vi "Read Data.vi"(3 "Error In":errorcluster) -> (0 "error out":errorcluster, 1 "text":string, 2 "appended path":path)   [LabVIEW 2017]
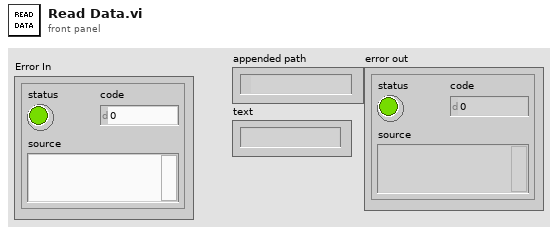
[diagram p1: front panel]
types:
  T1 = enum16{"open", "replace", "create", "open or create", "replace or create", "replace or create with confirmation"}
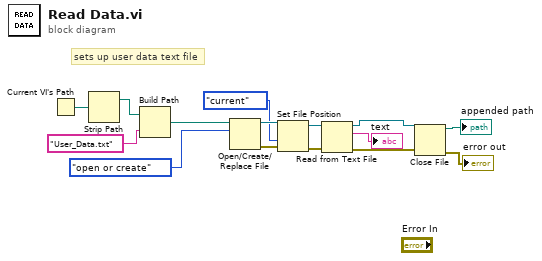
[diagram p0: block diagram]
diagram:
  # "sets up user data text file"
  n1 = Current VI's Path() -> (path=w8:path)
  n2 = Strip Path(path=w8) -> (stripped path=w14:path)  [unwired: 1 out]
  n3 = Build Path(base path=w14, name or relative path="User_Data.txt") -> (appended path=w12:path)
  n4 = Open/Create/Replace File(file path (use dialog)=w12, operation (0:open)=T1."open or create") -> (refnum out=w10:refnum<file>, error out=w11:errorcluster)  [unwired: 4 in, 1 out]
  n5 = Set File Position(refnum=w10, from (0:start)=enum16{"start", "end", "current"}."current", error in=w11) -> (refnum out=w6:refnum<file>, error out=w7:errorcluster)  [unwired: 1 in]
  n6 = Read from Text File(file (use dialog)=w6, error in=w7) -> (refnum out=w4:refnum<file>, text=→"text":string, error out=w3:errorcluster)  [unwired: 2 in, 1 out]
  n7 = Close File(refnum=w4, error in=w3) -> (path=→"appended path":path, error out=→"error out":errorcluster)
